vi "arduinoSerialComm.vi"() -> ()   [LabVIEW 2019]
uses:
  <vilib>/Instr/_visa.llb/VISA Configure Serial Port (Instr).vi
panel:
  in  "millisecond timer value":u32=1000
  in  "Ring":u16(ring)
  out "Recieve Log":string
  out "Serial Settings:Number of Bytes at Serial Port":u32
  in  "Turn On":bool
  in  "Turn Off":bool
  in  "Stop Button":bool
  in  "Baud Rate":u32=9600
  in  "COM Port":refnum<visa-resource-name>="COM4"
  out "Available?":bool
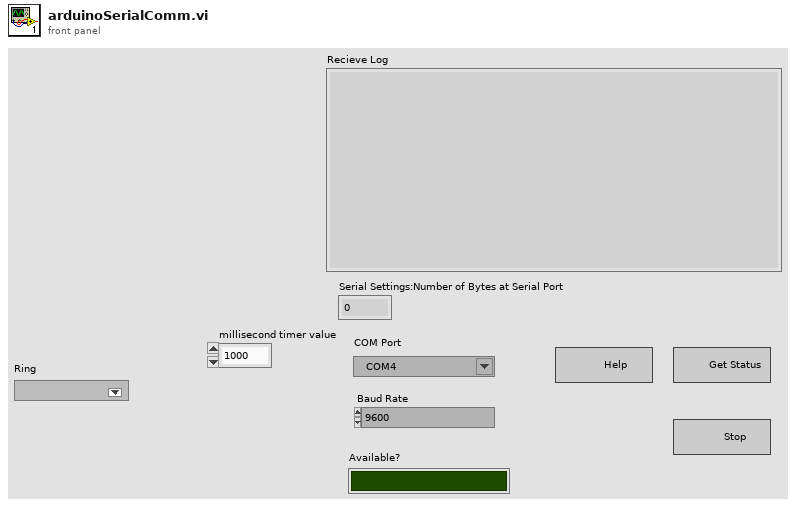
[diagram p1: front panel]
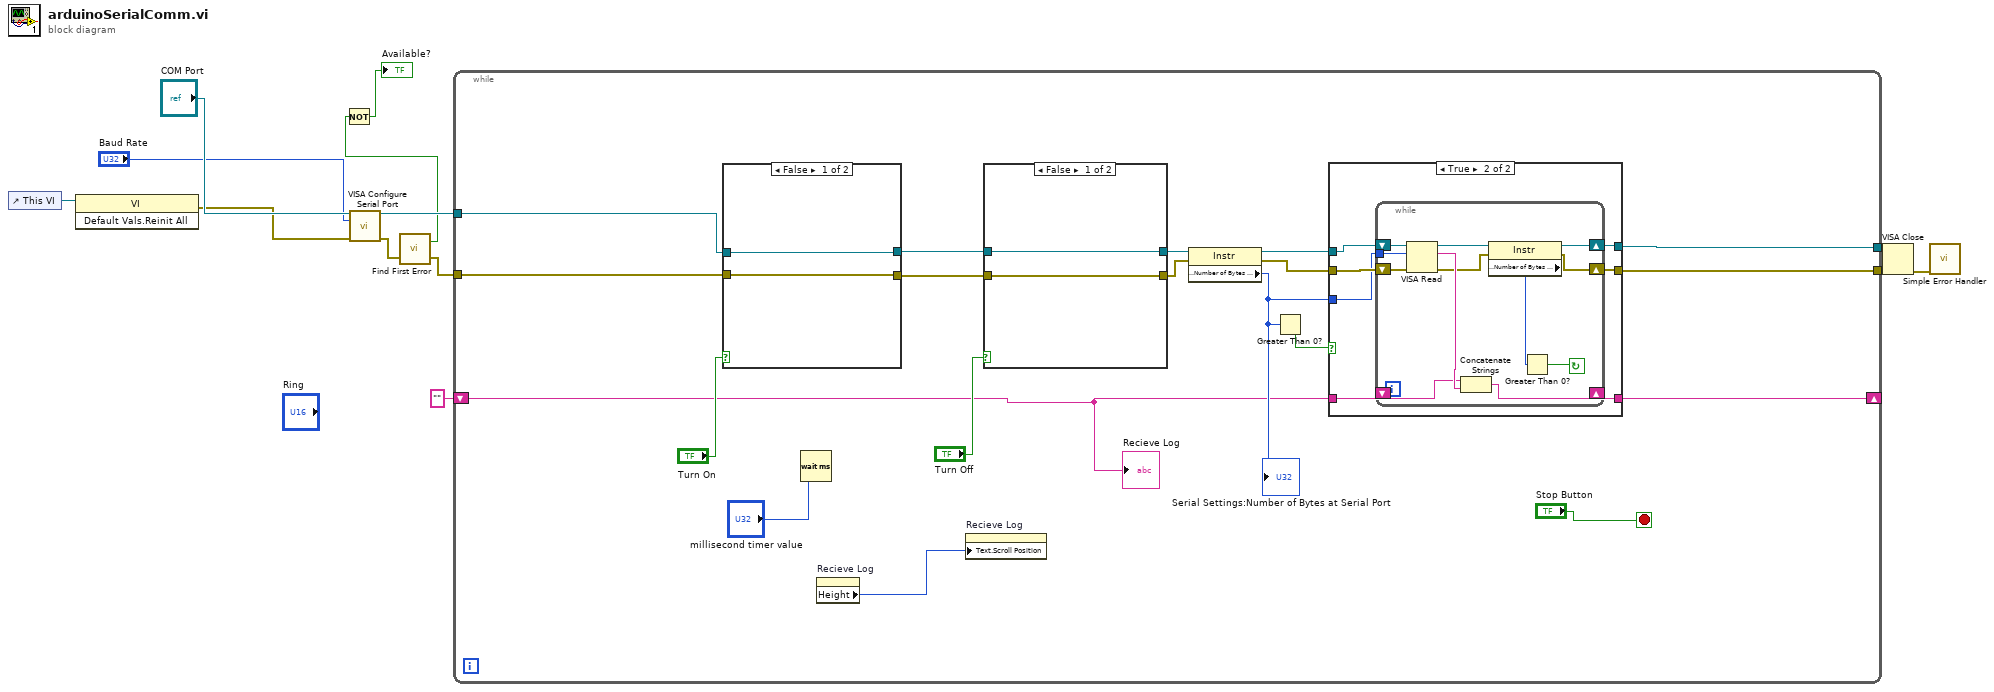
[diagram p0: block diagram]
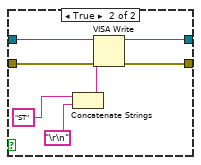
[diagram p3: hidden frame]
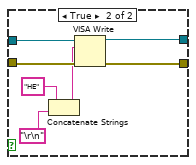
[diagram p4: hidden frame]
diagram:
  n1 = control-ref of="This VI"() -> (w10:refnum<vi>)
  n2 = invoke class="VI" method="Default Vals.Reinit All"(reference=w10) -> (error out=w6:errorcluster)  [unwired: 2 in, 2 out]
  n3 = call-poly "VISA Configure Serial Port"("VISA resource name"="COM Port", "baud rate (9600)"="Baud Rate", "error in (no error)"=w6) -> ("VISA resource name out"=w5:refnum<visa-resource-name>, "error out"=w4:errorcluster)  [unwired: 11 in]
  n4 = call <vilib>:"Find First Error.vi"("error in (no error)"=w4) -> ("error out"=w3:errorcluster, "error?"=w2:bool)  [unwired: 3 in]
  n5 = Not(x=w2) -> (.not. x?=→"Available?":bool)
  n6 = while {
    tunnel: [w25] -> w12
    tunnel: [w24] -> w13
    shift-right: [w18] -> _
    shift-left: "" -> [w14]
    tunnel: w5 -> [w16]
    tunnel: w3 -> [w15]
    stop <- "Stop Button" stop-if-true
    n7 = case shown="False" "Turn On" {
      tunnel: [w65 w72] -> w32
      tunnel: [w64 w71] -> w31
      tunnel: w16 -> [w65 w70]
      tunnel: w15 -> [w64 w69]
      frame False {
      }
      frame True {
        n8 = Concatenate Strings("HE" ("write buffer"), "\r\n") -> (w67:string)
        n9 = VISA Write(VISA resource name=w70, write buffer=w67, error in (no error)=w69) -> (VISA resource name out=w72:refnum<visa-resource-name>, error out=w71:errorcluster)  [unwired: 1 out]
      }
    }
    n10 = Wait (ms)(milliseconds to wait="millisecond timer value") -> ()  [unwired: 1 out]
    n11 = property on="Recieve Log" class="Str"() -> ("Height"=w17:u32)  [unwired: 2 in, 2 out]
    n12 = property on="Recieve Log" class="Str"("Text.Scroll Position"=w17) -> ()  [unwired: 2 in, 2 out]
    n13 = case shown="False" "Turn Off" {
      tunnel: w32 -> [w56 w63]
      tunnel: w31 -> [w55 w62]
      tunnel: [w55 w61] -> w29
      tunnel: [w56 w60] -> w30
      frame False {
      }
      frame True {
        n14 = Concatenate Strings("ST" ("write buffer"), "\r\n") -> (w59:string)
        n15 = VISA Write(VISA resource name=w63, write buffer=w59, error in (no error)=w62) -> (VISA resource name out=w60:refnum<visa-resource-name>, error out=w61:errorcluster)  [unwired: 1 out]
      }
    }
    n16 = property class="Instr"(reference=w30, error in=w29) -> (reference out=w26:refnum<visa-resource-name>, error out=w27:errorcluster, "Serial Settings:Number of Bytes at Serial Port"=w23:u32)
    "Serial Settings:Number of Bytes at Serial Port" <- w23
    n17 = Greater Than 0?(x=w23) -> (x > 0?=w28:bool)
    n18 = case shown="True" w28 {
      tunnel: w26 -> [w35 w42]
      tunnel: w27 -> [w34 w40]
      tunnel: [w35 w41] -> w25
      tunnel: [w34 w39] -> w24
      tunnel: w23 -> [_ w38]
      tunnel: w14 -> [w33 w37]
      tunnel: [w33 w36] -> w18
      frame False {
      }
      frame True {
        n19 = while {
          tunnel: w38 -> [w52]
          shift-right: [w43] -> w41
          shift-left: w42 -> [w54]
          shift-right: [w47] -> w39
          shift-left: w40 -> [w53]
          shift-right: [w49] -> w36
          shift-left: w37 -> [w50]
          stop <- w46 continue-if-true
          n20 = VISA Read(VISA resource name=w54, byte count=w52, error in (no error)=w53) -> (VISA resource name out=w44:refnum<visa-resource-name>, read buffer=w51:string, error out=w48:errorcluster)  [unwired: 1 out]
          n21 = Concatenate Strings(w50, w51) -> (w49:string)
          n22 = property class="Instr"(reference=w44, error in=w48) -> (reference out=w43:refnum<visa-resource-name>, error out=w47:errorcluster, "Serial Settings:Number of Bytes at Serial Port"=w45:u32)
          n23 = Greater Than 0?(x=w45) -> (x > 0?=w46:bool)
        }
      }
    }
    "Recieve Log" <- w14
  }
  n24 = VISA Close(VISA resource name=w12, error in (no error)=w13) -> (error out=w11:errorcluster)
  n25 = call <vilib>:"Simple Error Handler.vi"("error in (no error)"=w11) -> ()  [unwired: 4 in, 5 out]
